vi "from string.vi"(8 "error in":errorcluster, 9 "data":string, 10 "version":string, 11 "J1939 configuration in":refnum<class "J1939 configuration.lvclass">) -> (0 "error out":errorcluster, 3 "J1939 configuration out":refnum<class "J1939 configuration.lvclass">)   [LabVIEW 2013, in "J1939 configuration.lvclass"]
doc: "Provides an interface for loading a module configuration from a file or other serialized data source. It is recommended that all children of this class store data in two sets--data required for its own initialization, and any data required for parent initialization--and that each implementation uses the <b>Call Parent Method</b> primitive to de-serialize parent information. As a result, it is expected that every module configuration class calls <b>component configuration.lvclass:From String.vi</b>."
uses:
  J1939 configuration.lvclass
  XNET Settings.ctl
  <vilib>/NI/Tag Bus Module Framework/module configuration/TBM module configuration.lvclass
  <vilib>/NI/Tag Bus Module Framework/channel/TBM channel.lvclass
  Line.ctl
  J1939 configuration.lvclass/J1939 configuration.ctl
  <vilib>/NI/Configuration Framework/serializable configuration/NISE_CEF_serializable configuration.lvclass
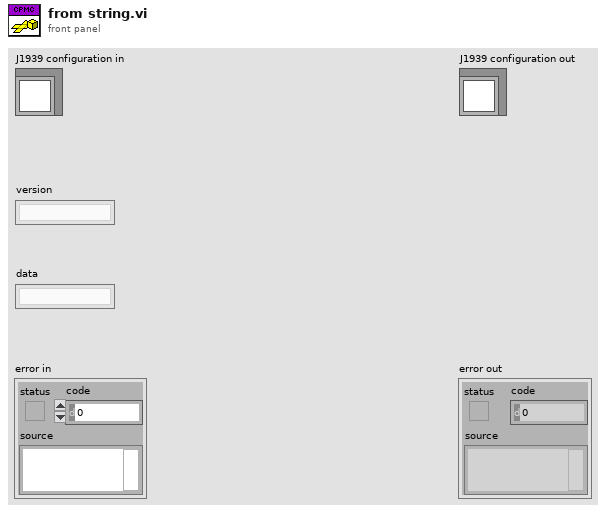
[diagram p1: front panel]
types:
  T1 = typedef "J1939 configuration.lvclass/XNET Settings.ctl" = cluster{"Select Interface":refnum<k21>, "Node Address":u8, "Node Name":u64}
  T2 = typedef "J1939 configuration.lvclass/Line.ctl" = cluster{"channel":refnum<class "TBM channel.lvclass">, "XNET Signal":refnum<k21>}
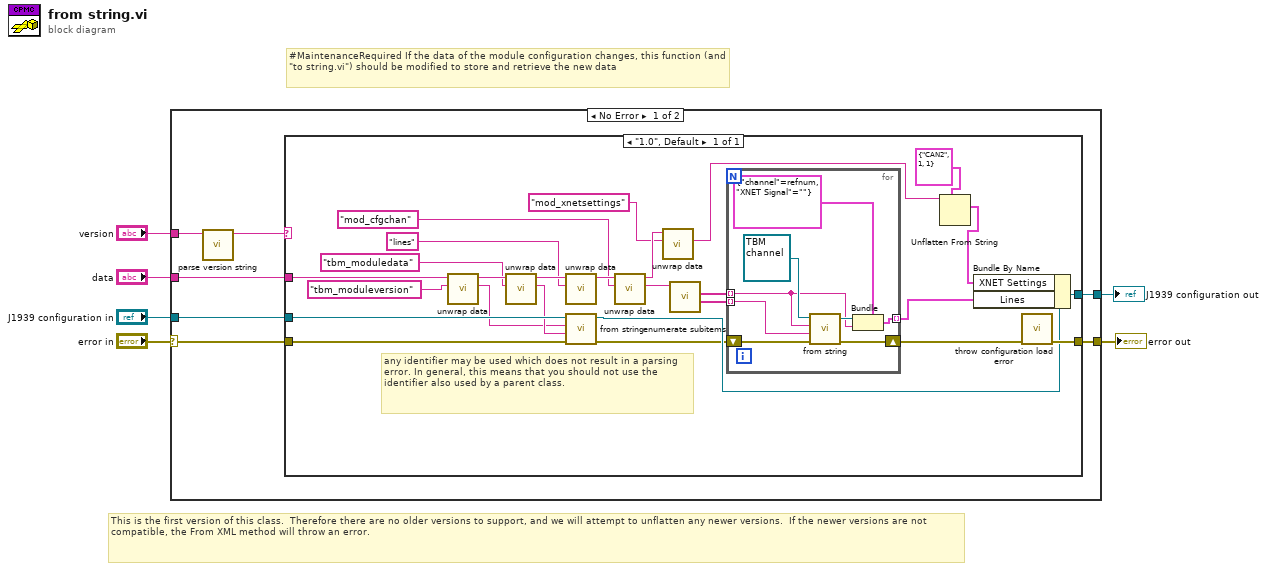
[diagram p0: block diagram]
diagram:
  # "#MaintenanceRequired If the data of the module configuration changes, this function (and \"to string.vi\") should be modified to store and retrieve the new data"
  # "This is the first version of this class.  Therefore there are no older versions to support, and we will attempt to unflatten any newer versions.  If the newer versions are not compatible, the From XML method will throw an error."
  n1 = case shown="No Error" "error in" {
    selector: "error in" -> [w7 w49]
    tunnel: "data" -> [w13 _]
    tunnel: "J1939 configuration in" -> [w12 w48]
    tunnel: [w11 w48] -> w5
    tunnel: [w10 w49] -> w4
    tunnel: "version" -> [w9 _]
    frame No Error {
      n2 = call <vilib>:"parse version string.vi"("full version"=w9) -> ("major.minor version"=w8:string)  [unwired: 7 in, 3 out]
      n3 = case shown="\"1.0\", Default" w8 {
        tunnel: w13 -> [w36]
        tunnel: w7 -> [w35]
        tunnel: w12 -> [w39]
        tunnel: [w27] -> w11
        tunnel: [w38] -> w10
        frame "1.0", Default {
          # "any identifier may be used which does not result in a parsing error. In general, this means that you should not use the identifier also used by a parent class."
          n4 = call <vilib>:"unwrap data.vi"("identifier"="tbm_moduleversion" ("additional identifier"), "data to unwrap"=w36) -> ("unwrapped data"=w31:string, "remaining string"=w37:string)  [unwired: 8 in]
          n5 = call <vilib>:"unwrap data.vi"("identifier"="tbm_moduledata" ("additional identifier"), "data to unwrap"=w37) -> ("unwrapped data"=w33:string, "remaining string"=w30:string)  [unwired: 8 in]
          n6 = call <vilib>:"unwrap data.vi"("identifier"="lines" ("additional identifier"), "data to unwrap"=w30) -> ("remaining string"=w26:string)  [unwired: 8 in, 1 out]
          n7 = call-parent "from string.vi"("error in"=w35, "data"=w33, "version"=w31, "module configuration in"=w39) -> ("error out"=w22:errorcluster, "module configuration out"=w28:refnum<class "J1939 configuration.lvclass">)  [unwired: 6 in]
          n8 = call <vilib>:"unwrap data.vi"("identifier"="mod_cfgchan", "data to unwrap"=w26) -> ("unwrapped data"=w21:string, "remaining string"=w18:string)  [unwired: 8 in]
          n9 = call <vilib>:"unwrap data.vi"("identifier"="mod_xnetsettings", "data to unwrap"=w18) -> ("unwrapped data"=w16:string)  [unwired: 8 in, 1 out]
          n10 = call <vilib>:"enumerate subitems.vi"("data to enumerate"=w21) -> ("associated data"=w23:string[], "discovered subitems"=w24:string[])  [unwired: 8 in, 1 out]
          n11 = for {
            shift-right: [w47] -> w19
            shift-left: w22 -> [w46]
            tunnel: w24 -> [w40] mode=indexing
            tunnel: w23 -> [w45] mode=indexing
            tunnel: [w41] -> w20 mode=indexing
            n12 = call-dynamic "from string.vi"("error in"=w46, "channel data"=w45, "identifier"=w40, "channel in"=refnum<class "TBM channel.lvclass"> refnum) -> ("error out"=w47:errorcluster, "channel out"=w42:refnum<class "TBM channel.lvclass">)  [unwired: 6 in]
            n13 = Bundle(cluster=T2 {"channel"=refnum, "XNET Signal"=""} ("Line"), "channel"=w42, "XNET Signal"=w40) -> (w41:T2)
          }
          n14 = Unflatten From String(type=T1 {"Select Interface"="CAN2", "Node Address"=1, "Node Name"=1} ("XNET Settings"), binary string=w16) -> (value=w14:T1)  [unwired: 3 in, 2 out]
          n15 = Bundle By Name(cluster=w28, "XNET Settings"=w14, "Lines"=w20) -> (w27:refnum<class "J1939 configuration.lvclass">)
          n16 = call <vilib>:"throw configuration load error.vi"("error in"=w19) -> ("error out"=w38:errorcluster)  [unwired: 10 in]
        }
      }
    }
    frame Error {
    }
  }
  "error out" <- w4
  "J1939 configuration out" <- w5
